vi "MListbox Init.vi"(0 "Multicolumn ListBox in":refnum<class "Multicolumn ListBox.lvclass">, 1 "Header Backcolor":u32(colorbox)=16448250, 3 "Select Entire Rows":bool=TRUE, 5 "MListbox Ref":refnum<vi>, 9 "Row Backcolor":u32[](array[colorbox])=[16448250], 11 "error in (no error)":errorcluster, 12 "RowNumDisplay":u16, 14 "Initialize":cluster{"Row":u16, "Colunm":u16}) -> (4 "Multicolumn ListBox out":refnum<class "Multicolumn ListBox.lvclass">, 15 "error out":errorcluster)   [LabVIEW 2018, in "Multicolumn ListBox.lvclass"]
uses:
  Multicolumn ListBox.lvclass
  Multicolumn ListBox.lvclass/Multicolumn ListBox.ctl
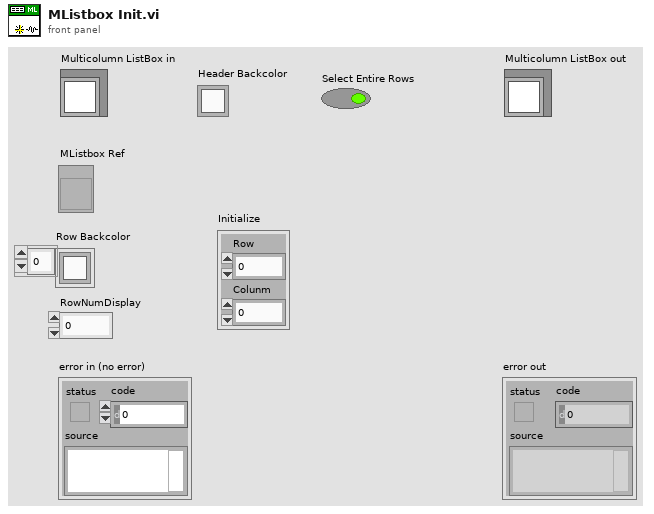
[diagram p1: front panel]
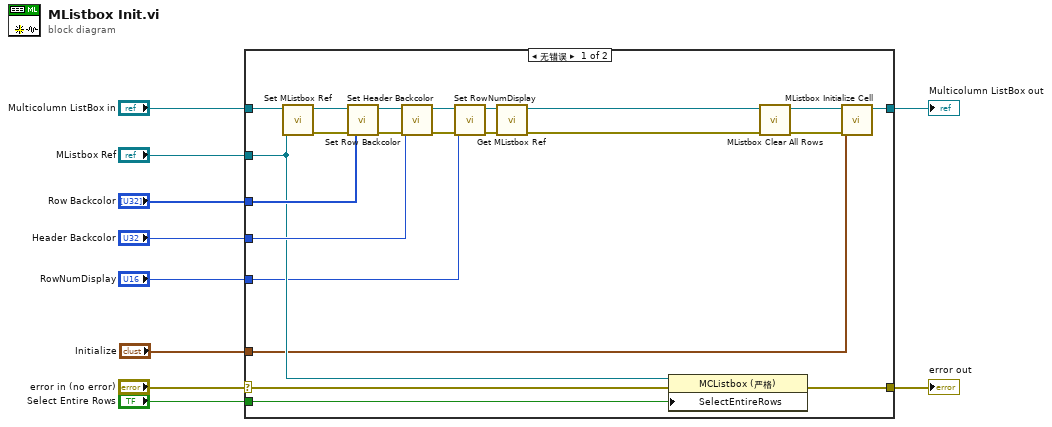
[diagram p0: block diagram]
diagram:
  n1 = case shown="无错误" "error in (no error)" {
    selector: "error in (no error)" -> [w25 w34]
    tunnel: [w24 w34] -> w9
    tunnel: [w20 w33] -> w7
    tunnel: "Multicolumn ListBox in" -> [w31 w33]
    tunnel: "MListbox Ref" -> [w26 _]
    tunnel: "Row Backcolor" -> [w30 _]
    tunnel: "Header Backcolor" -> [w27 _]
    tunnel: "Select Entire Rows" -> [w23 _]
    tunnel: "RowNumDisplay" -> [w22 _]
    tunnel: "Initialize" -> [w19 _]
    frame No Error {
      n2 = call "Set MListbox Ref.vi"("MListbox Ref"=w26, "Multicolumn ListBox in"=w31) -> ("error out"=w16:errorcluster, "Multicolumn ListBox out"=w32:refnum<class "Multicolumn ListBox.lvclass">)  [unwired: 8 in]
      n3 = call "Set Row Backcolor.vi"("error in (no error)"=w16, "Row Backcolor"=w30, "Multicolumn ListBox in"=w32) -> ("error out"=w15:errorcluster, "Multicolumn ListBox out"=w29:refnum<class "Multicolumn ListBox.lvclass">)  [unwired: 7 in]
      n4 = call "Set Header Backcolor.vi"("error in (no error)"=w15, "Header Backcolor"=w27, "Multicolumn ListBox in"=w29) -> ("error out"=w14:errorcluster, "Multicolumn ListBox out"=w28:refnum<class "Multicolumn ListBox.lvclass">)  [unwired: 7 in]
      n5 = call "Set RowNumDisplay.vi"("error in (no error)"=w14, "RowNumDisplay"=w22, "Multicolumn ListBox in"=w28) -> ("error out"=w17:errorcluster, "Multicolumn ListBox out"=w18:refnum<class "Multicolumn ListBox.lvclass">)  [unwired: 7 in]
      n6 = call "Get MListbox Ref.vi"("error in (no error)"=w17, "Multicolumn ListBox in"=w18) -> ("error out"=w13:errorcluster, "Multicolumn ListBox out"=w11:refnum<class "Multicolumn ListBox.lvclass">)  [unwired: 7 in, 1 out]
      n7 = property class="MCListbox (严格)"(reference=w26, error in=w25, "SelectEntireRows"=w23) -> (error out=w24:errorcluster)  [unwired: 1 out]
      n8 = call "MListbox Clear All Rows.vi"("error in (no error)"=w13, "Multicolumn ListBox in"=w11) -> ("error out"=w12:errorcluster, "Multicolumn ListBox out"=w21:refnum<class "Multicolumn ListBox.lvclass">)  [unwired: 8 in]
      n9 = call "MListbox Initialize Cell.vi"("error in (no error)"=w12, "Initialize"=w19, "Multicolumn ListBox in"=w21) -> ("Multicolumn ListBox out"=w20:refnum<class "Multicolumn ListBox.lvclass">)  [unwired: 7 in, 1 out]
    }
    frame Error {
    }
  }
  "error out" <- w9
  "Multicolumn ListBox out" <- w7
